vi "Handle Message.vi"(8 "error in (no error)":errorcluster, 9 "Message Completion Handler":refnum<class "Message Completion Handler.lvclass">, 10 "Message":string, 11 "Sift TDMS Uploader in":refnum<class "Sift TDMS Uploader.lvclass">) -> (0 "error out":errorcluster, 1 "Synchronously Complete Message?":bool=TRUE, 2 "Message Response":string, 3 "Sift TDMS Uploader out":refnum<class "Sift TDMS Uploader.lvclass">)   [LabVIEW 2024, in "Sift TDMS Uploader.lvlib" / "Sift TDMS Uploader.lvclass"]
uses:
  Sift TDMS Uploader.lvclass
  C:/Program Files/National Instruments/LabVIEW 2024/vi.lib/FlexLogger/SDK/PluginSDK.lvlibp/PEFClasses/SDK/Processing Element/Processing Element.lvclass
  <vilib>/FlexLogger/SDK/PluginSDK.lvlibp/PEFClasses/SDK/Message Completion Handler/Message Completion Handler.lvclass
  Sift TDMS Uploader.lvclass/Sift TDMS Uploader.ctl
  Globals.vi
  <vilib>/FlexLogger/SDK/PluginSDK.lvlibp/PEFClasses/SDK/Processing Element/Read System Interface.vi
  <vilib>/FlexLogger/SDK/PluginSDK.lvlibp/PEFClasses/SDK/Processing Element/Read Alias.vi
  <vilib>/FlexLogger/SDK/PluginSDK.lvlibp/PEFClasses/SDK/System Interface/System Interface.lvclass
  <vilib>/FlexLogger/SDK/PluginSDK.lvlibp/PEFClasses/SDK/Plugin/Plugin.lvclass
  C:/Program Files/National Instruments/LabVIEW 2024/vi.lib/FlexLogger/SDK/PluginSDK.lvlibp/PEFClasses/SDK/Plugin/Plugin.lvclass
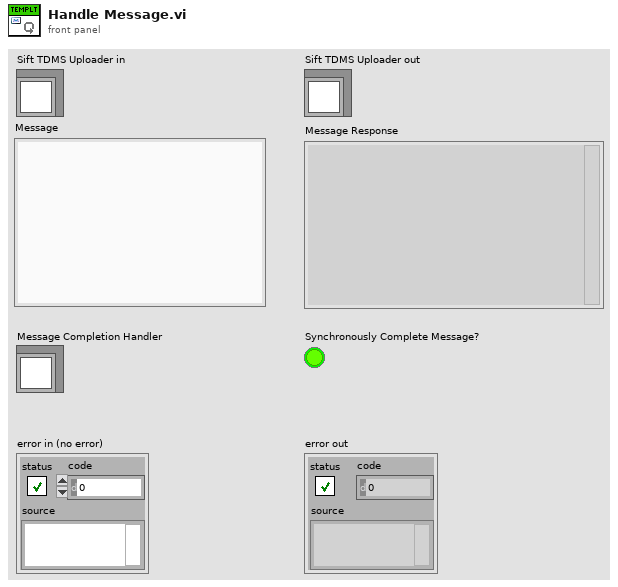
[diagram p1: front panel]
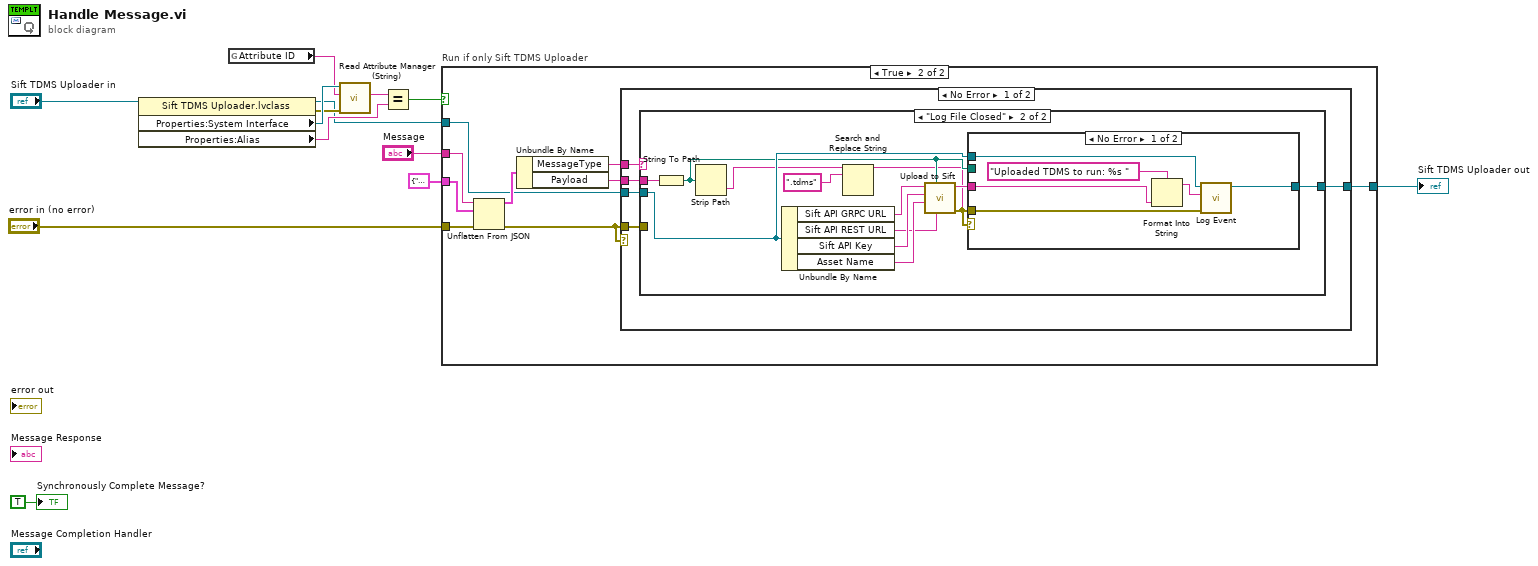
[diagram p0: block diagram]
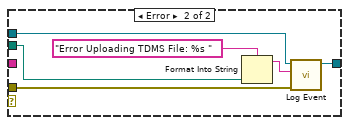
[diagram p4: hidden frame]
diagram:
  n1 = property class="Sift TDMS Uploader.lvclass"(reference="Sift TDMS Uploader in") -> (reference out=w1:refnum<class "Sift TDMS Uploader.lvclass">, error out=w11:errorcluster, "Properties:System Interface"=w12:refnum<class "System Interface.lvclass">, "Properties:Alias"=w3:string)  [unwired: 1 in]
  n2 = global read "Globals.vi" "Attribute ID"() -> (w10:string)
  n3 = call-dynamic "Read Attribute Manager (String).vi"("error in (no error)"=w11, "Attribute ID"=w10, "System Interface in"=w12) -> ("Attrib Val"=w4:string)  [unwired: 5 in, 3 out]
  n4 = Equal?(x=w4, y=w3) -> (x = y?=w9:bool)
  n5 = case "Run if only Sift TDMS Uploader" shown="True" w9 {
    tunnel: w1 -> [w14 w19]
    tunnel: "Message" -> [_ w18]
    tunnel: cluster{"Payload":string, "MessageType":string} {"Payload"="", "MessageType"=""} -> [_ w17]
    tunnel: "error in (no error)" -> [_ w16]
    tunnel: [w14 w15] -> w5
    frame False {
    }
    frame True {
      n6 = Unflatten From JSON(JSON string=w18, type and defaults=w17, error in (no error)=w16) -> (value=w20:cluster{"Payload":string, "MessageType":string}, error out=w21:errorcluster)  [unwired: 4 in]
      n7 = Unbundle By Name(w20) -> ("MessageType"=w22:string, "Payload"=w23:string)
      n8 = case shown="No Error" w21 {
        tunnel: w22 -> [w28 _]
        tunnel: w23 -> [w26 _]
        tunnel: w19 -> [w27 w55]
        tunnel: [w24 w55] -> w15
        tunnel: w21 -> [w25 _]
        frame No Error {
          n9 = case shown="\"Log File Closed\"" w28 {
            tunnel: w26 -> [_ w42]
            tunnel: w27 -> [w29 w37]
            tunnel: [w29 w36] -> w24
            tunnel: w25 -> [_ _]
            frame Default {
            }
            frame "Log File Closed" {
              n10 = String To Path(string=w42) -> (path=w35:path)
              n11 = Strip Path(path=w35) -> (name=w31:string)  [unwired: 1 out]
              n12 = Unbundle By Name(w37) -> ("Sift API GRPC URL"=w41:string, "Sift API REST URL"=w38:string, "Sift API Key"=w40:string, "Asset Name"=w39:string)
              n13 = Search and Replace String(input string=w31, search string=".tdms") -> (result string=w32:string)  [unwired: 6 in, 3 out]
              n14 = call "Upload to Sift.vi"("API REST URL"=w38, "Absolute Filepath"=w35, "Run Name"=w32, "Asset Name"=w39, "API Key"=w40, "API GRPC URL"=w41) -> ("Error"=w33:errorcluster, "Run URL"=w34:string)  [unwired: 4 in]
              n15 = case shown="No Error" w33 {
                tunnel: w33 -> [w47 w54]
                tunnel: w37 -> [w48 w53]
                tunnel: [w46 w52] -> w36
                tunnel: w35 -> [_ w51]
                tunnel: w34 -> [w43 _]
                frame No Error {
                  n16 = Format Into String(format string="Uploaded TDMS to run: %s ", w43) -> (resulting string=w44:string)  [unwired: 2 in, 1 out]
                  n17 = call <vilib>:"Log Event.vi"("error in (no error)"=w47, "Message"=w44, "Plugin in"=w48) -> ("Plugin out"=w46:refnum<class "Sift TDMS Uploader.lvclass">)  [unwired: 7 in, 1 out]
                }
                frame Error {
                  n18 = Format Into String(format string="Error Uploading TDMS File: %s ", w51) -> (resulting string=w49:string)  [unwired: 2 in, 1 out]
                  n19 = call <vilib>:"Log Event.vi"("error in (no error)"=w54, "Message"=w49, "Plugin in"=w53) -> ("Plugin out"=w52:refnum<class "Sift TDMS Uploader.lvclass">)  [unwired: 7 in, 1 out]
                }
              }
            }
          }
        }
        frame Error {
        }
      }
    }
  }
  "Sift TDMS Uploader out" <- w5
  "Synchronously Complete Message?" <- TRUE ("Synchronously Complete Message?")
